vi "Translator.vi"(0 "Input":variant, 11 "error in (no error)":errorcluster) -> (4 "Output":variant, 15 "error out":errorcluster)   [LabVIEW 2014, in "Arduino MatrixMath.lvlib"]
doc: "An example of how to create the Translator to convert the LabVIEW VIs to Arduino C code."
uses:
  <vilib>/Aledyne-TSXperts/Arduino Compatible Compiler for LabVIEW/addons/Arduino MatrixMath/Arduino MatrixMath.lvlib
panel:
  out "Outputs":string[](array[string])
  out "Inputs":string[](array[string])
  out "Output Datatypes":string[](array[string])
  out "Input Datatypes":string[](array[string])
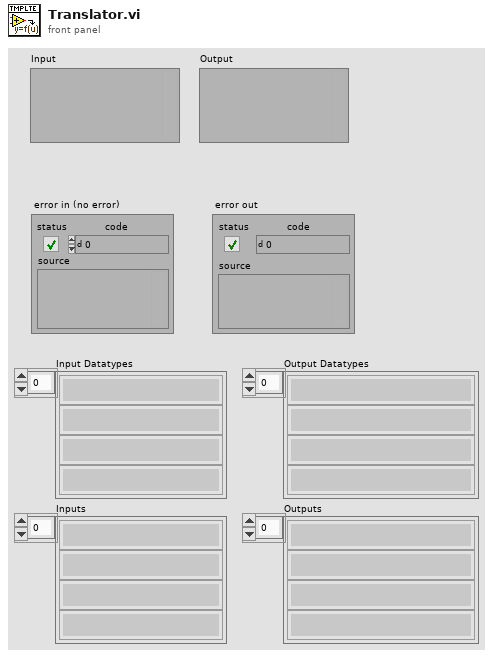
[diagram p1: front panel]
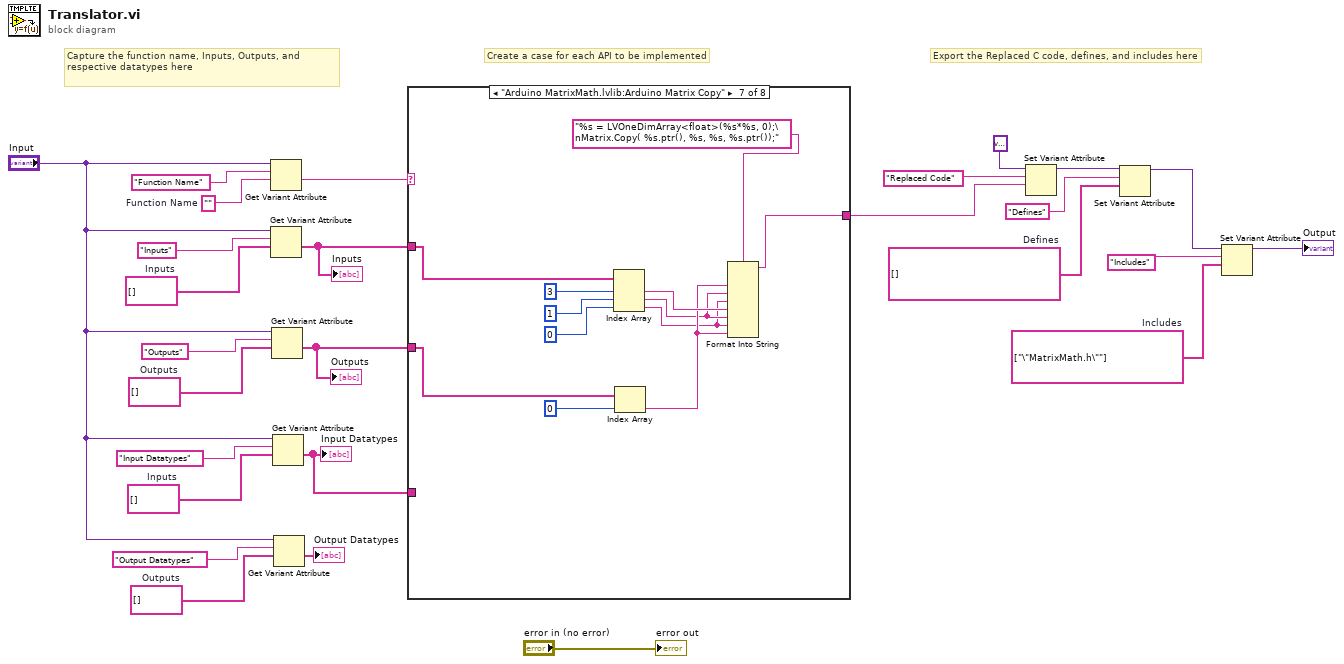
[diagram p0: block diagram]
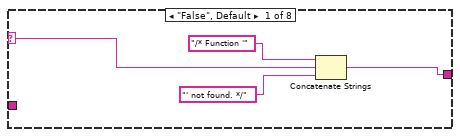
[diagram p2: hidden frame]
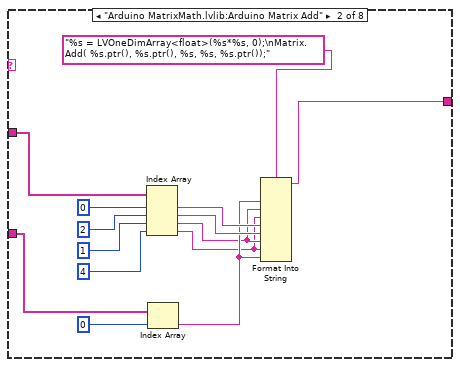
[diagram p3: hidden frame]
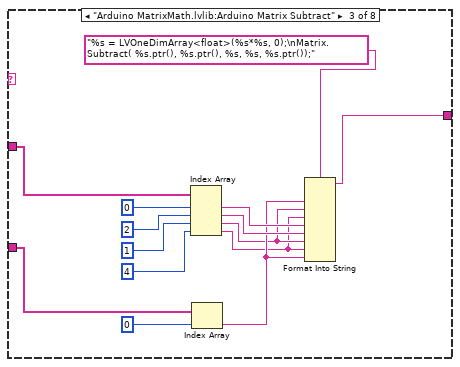
[diagram p4: hidden frame]
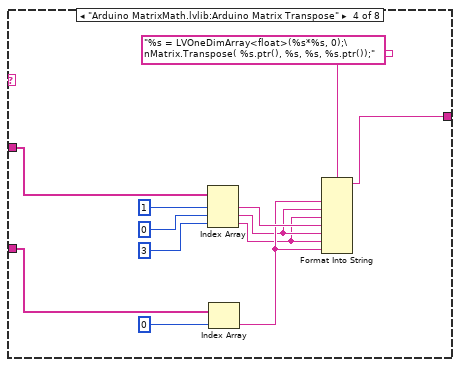
[diagram p5: hidden frame]
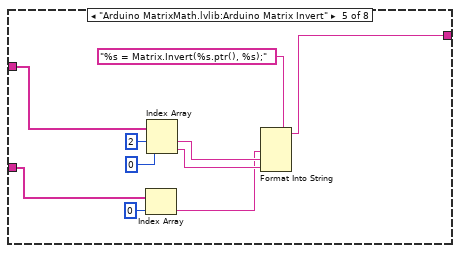
[diagram p6: hidden frame]
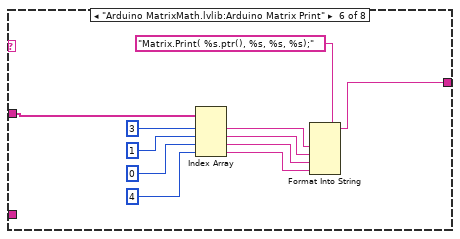
[diagram p7: hidden frame]
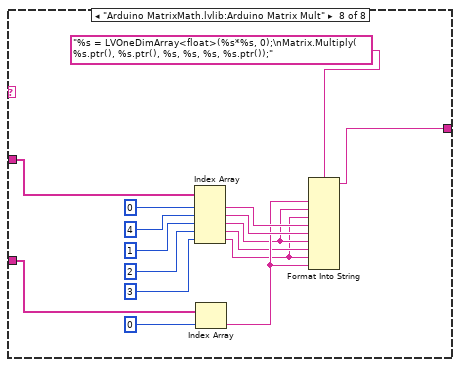
[diagram p8: hidden frame]
diagram:
  w2 = string[] []  # Defines
  w12 = string[] []  # Outputs
  w13 = string[] []  # Inputs
  w18 = string[] ["\"MatrixMath.h\""]  # Includes
  w23 = string[] []  # Outputs
  w24 = string[] []  # Inputs
  w25 = ""  # Function Name
  # "Capture the function name, Inputs, Outputs, and respective datatypes here"
  # "Export the Replaced C code, defines, and includes here"
  # "Create a case for each API to be implemented"
  n1 = Get Variant Attribute(Variant="Input", name="Function Name", default value (empty Variant)=w25) -> (value=w20:string)  [unwired: 1 in, 3 out]
  n2 = Get Variant Attribute(Variant="Input", name="Inputs", default value (empty Variant)=w24) -> (value=w7:string[])  [unwired: 1 in, 3 out]
  "Inputs" <- w7
  n3 = Get Variant Attribute(Variant="Input", name="Outputs", default value (empty Variant)=w23) -> (value=w8:string[])  [unwired: 1 in, 3 out]
  "Outputs" <- w8
  n4 = Get Variant Attribute(Variant="Input", name="Input Datatypes", default value (empty Variant)=w13) -> (value=w1:string[])  [unwired: 1 in, 3 out]
  "Input Datatypes" <- w1
  n5 = Get Variant Attribute(Variant="Input", name="Output Datatypes", default value (empty Variant)=w12) -> (value=→"Output Datatypes":string[])  [unwired: 1 in, 3 out]
  n6 = case shown="\"Arduino MatrixMath.lvlib:Arduino Matrix Copy\"" w20 {
    selector: w20 -> [w30 _ _ _ _ _ _ _]
    tunnel: [w28 w42 w49 w63 w78 w82 w96 w112] -> w19
    tunnel: w7 -> [_ w45 w51 w65 w81 w83 w98 w111]
    tunnel: w8 -> [_ w37 w50 w64 w73 _ w97 w110]
    tunnel: w1 -> [_ _ _ _ _ _ _ _]
    frame "False", Default {
      n7 = Concatenate Strings("/* Function '", w30, "' not found. */") -> (w28:string)
    }
    frame "Arduino MatrixMath.lvlib:Arduino Matrix Add" {
      n8 = Index Array(array=w45, index #1=0 ("index"), index #2=2 ("index"), index #3=1 ("index"), index #4=4 ("index")) -> (element #1=w41:string, element #2=w40:string, element #3=w33:string, element #4=w32:string)
      n9 = Index Array(array=w37, index=0) -> (element=w34:string)
      n10 = Format Into String(format string="%s = LVOneDimArray<float>(%s*%s, 0);\nMatrix.Add( %s.ptr(), %s.ptr(), %s, %s, %s.ptr());", w34, w33, w32, w41, w40, w33, w32, w34) -> (resulting string=w42:string)  [unwired: 2 in, 1 out]
    }
    frame "Arduino MatrixMath.lvlib:Arduino Matrix Subtract" {
      n11 = Index Array(array=w51, index #1=0 ("index"), index #2=2 ("index"), index #3=1 ("index"), index #4=4 ("index")) -> (element #1=w57:string, element #2=w56:string, element #3=w47:string, element #4=w46:string)
      n12 = Index Array(array=w50, index=0) -> (element=w48:string)
      n13 = Format Into String(format string="%s = LVOneDimArray<float>(%s*%s, 0);\nMatrix.Subtract( %s.ptr(), %s.ptr(), %s, %s, %s.ptr());", w48, w47, w46, w57, w56, w47, w46, w48) -> (resulting string=w49:string)  [unwired: 2 in, 1 out]
    }
    frame "Arduino MatrixMath.lvlib:Arduino Matrix Transpose" {
      n14 = Index Array(array=w65, index #1=1 ("index"), index #2=0 ("index"), index #3=3 ("index")) -> (element #1=w69:string, element #2=w61:string, element #3=w60:string)
      n15 = Index Array(array=w64, index=0) -> (element=w62:string)
      n16 = Format Into String(format string="%s = LVOneDimArray<float>(%s*%s, 0);\nMatrix.Transpose( %s.ptr(), %s, %s, %s.ptr());", w62, w61, w60, w69, w61, w60, w62) -> (resulting string=w63:string)  [unwired: 2 in, 1 out]
    }
    frame "Arduino MatrixMath.lvlib:Arduino Matrix Invert" {
      n17 = Index Array(array=w73, index=0) -> (element=w72:string)
      n18 = Index Array(array=w81, index #1=2 ("index"), index #2=0 ("index")) -> (element #1=w77:string, element #2=w75:string)
      n19 = Format Into String(format string="%s = Matrix.Invert(%s.ptr(), %s);", w72, w77, w75) -> (resulting string=w78:string)  [unwired: 2 in, 1 out]
    }
    frame "Arduino MatrixMath.lvlib:Arduino Matrix Print" {
      n20 = Index Array(array=w83, index #1=3 ("index"), index #2=1 ("index"), index #3=0 ("index"), index #4=4 ("index")) -> (element #1=w90:string, element #2=w86:string, element #3=w85:string, element #4=w84:string)
      n21 = Format Into String(format string="Matrix.Print( %s.ptr(), %s, %s, %s);", w90, w86, w85, w84) -> (resulting string=w82:string)  [unwired: 2 in, 1 out]
    }
    frame "Arduino MatrixMath.lvlib:Arduino Matrix Copy" {
      n22 = Index Array(array=w98, index #1=3 ("index"), index #2=1 ("index"), index #3=0 ("index")) -> (element #1=w102:string, element #2=w94:string, element #3=w93:string)
      n23 = Index Array(array=w97, index=0) -> (element=w95:string)
      n24 = Format Into String(format string="%s = LVOneDimArray<float>(%s*%s, 0);\nMatrix.Copy( %s.ptr(), %s, %s, %s.ptr());", w95, w94, w93, w102, w94, w93, w95) -> (resulting string=w96:string)  [unwired: 2 in, 1 out]
    }
    frame "Arduino MatrixMath.lvlib:Arduino Matrix Mult" {
      n25 = Index Array(array=w111, index #1=0 ("index"), index #2=4 ("index"), index #3=1 ("index"), index #4=2 ("index"), index #5=3 ("index")) -> (element #1=w118:string, element #2=w117:string, element #3=w107:string, element #4=w106:string, element #5=w105:string)
      n26 = Index Array(array=w110, index=0) -> (element=w108:string)
      n27 = Format Into String(format string="%s = LVOneDimArray<float>(%s*%s, 0);\nMatrix.Multiply( %s.ptr(), %s.ptr(), %s, %s, %s, %s.ptr());", w108, w107, w105, w118, w117, w107, w106, w105, w108) -> (resulting string=w112:string)  [unwired: 2 in, 1 out]
    }
  }
  n28 = Set Variant Attribute(Variant=variant ("variant"), name="Replaced Code", value=w19) -> (Variant out=w5:variant)  [unwired: 1 in, 2 out]
  n29 = Set Variant Attribute(Variant=w5, name="Defines", value=w2) -> (Variant out=w4:variant)  [unwired: 1 in, 2 out]
  n30 = Set Variant Attribute(Variant=w4, name="Includes", value=w18) -> (Variant out=→"Output":variant)  [unwired: 1 in, 2 out]
  "error out" <- "error in (no error)"
